vi "CV.vi"(2 "Run uninterrupted?":bool, 3 "Device Category IN:":string(combo)="ATLAS18SS" caption="Device Category:", 4 "Batch No. IN:":string caption="Batch No.:", 5 "Wafer No. IN:":string caption="Wafer No.:", 6 "DB Serial No. IN:":string caption="DB Serial No.:") -> (0 "Done!":bool)   [LabVIEW 2013]
doc: "Performs CV measurements according to ATLAS ITk Quality Control Specifications."
uses:
  InstrControl/Switching/Switching.lvclass
  InstrControl/SupplyControl/SupplyControl.lvclass
  InstrControl/LCRControl/LCRControl.lvclass
  general_VIs/globals/QC_MeasurementSetup.vi
  general_VIs/globals/QC_RunInformation.vi
  InstrControl/InstrumentSetup.vi
  InstrControl/ArduinoControl/ArduinoControl.lvclass
  <vilib>/Analysis/NI_AALBase.lvlib
  InstrControl/InstrControl.lvclass
panel:
  out "Tab Control 2":enum32{"CV Setup", "CV Scan"}(tab)
  in  "V_depletion limit [V]":dbl=-300.0
  in  "step interval [s] IN":i32=5 caption="step interval [s]"
  in  "step [V] IN":dbl=10.0 caption="step [V]" format="%.1f"
  in  "Final volts [V] IN":dbl=-500.0 caption="Final volts [V]"
  in  "Initial volts [V] IN":dbl caption="Initial volts [V]"
  in  "Current Limit [µA]":dbl=1000.0 min=0.0001 format="%.3f"
  in  "Continue":bool
  in  "Quit":bool
  in  "Software current limit?":bool
  in  "Frequency [Hz] Setup":i32=500 caption="Frequency [Hz]" format="%#.3p"
  in  "Measurement Configurations":bool
  out "RH":dbl[](array[numeric]) caption="RH [%]" format="%#.2f"
  out "step interval [s]":u32=5
  out "step [V]":dbl=10.0 format="%.1f"
  out "Final volts [V]":dbl=-700.0 format="%.1f"
  out "Initial volts [V]":dbl format="%.1f"
  out "Frequency [Hz]":i32=1000 format="%#.3p"
  out "Temp.":dbl[](array[numeric]) caption="Temp. [°C]" format="%#.2f"
  out "Volts":dbl[](array[numeric]) caption="Volts [V]"
  out "Resistance":dbl[](array[numeric]) caption="Res [kOhm]"
  out "Capacitance":dbl[](array[numeric]) caption="Cap [pF]"
  out "Cgraph":cluster{"Initial volts":dbl, dbl, dbl[]}(graph)
  in  "Scales":T1(ring)
  in  "Cscale":enum16{"1/C^2 [1/nF^2]", "nF", "pF"}(ring)
  out "positive ramp?":bool
  out "Tab Control":enum32{"CV Setup", "CV Scan"}(tab)
  in  "LCR Meter":string(combo)="WayneKerr 6440B"
  in  "User:":string(combo)="Christoph"
  in  "CV Supply":string(combo)="Keithley 2410"
  in  "Hardware Configurations":bool
  in  "Temperature":enum16{"Read Arduino", "Enter manually"}(ring)
  in  "Manufacturer:":string(combo)="Hamamatsu"
  in  "abort":bool
  out "Device Category:":string
  out "DB Serial No.:":string
  out "Current Volts:":dbl format="%.2f"
  in  "quit (no save)":bool
  in  "Quit & Save":bool
  out "Bias On/Off:":bool
  out "STATUS 1":string
  out "Initiated:":string
  out "Sensor No.:":string
  out "No of steps":u32
  out "Current reading No.":u32
  out "Last reading at:":string
  in  "Simulation":bool
  # "Strip Sensor QC: CV"
  # "University of\nCambridge"
  # "Vertical Scale:"
  # "Measurement Configuration"
  # "CV Scan parameters:"
  # "Last 5 readings:"
  # "n-4"
  # "n-3"
  # "n-2"
  # "n-1"
  # "n"
  # "DUT Description"
  # "Hardware"
  # "DUT & Test Description:"
  # "Current status:"
  # "Rdg No:"
  # "out of"
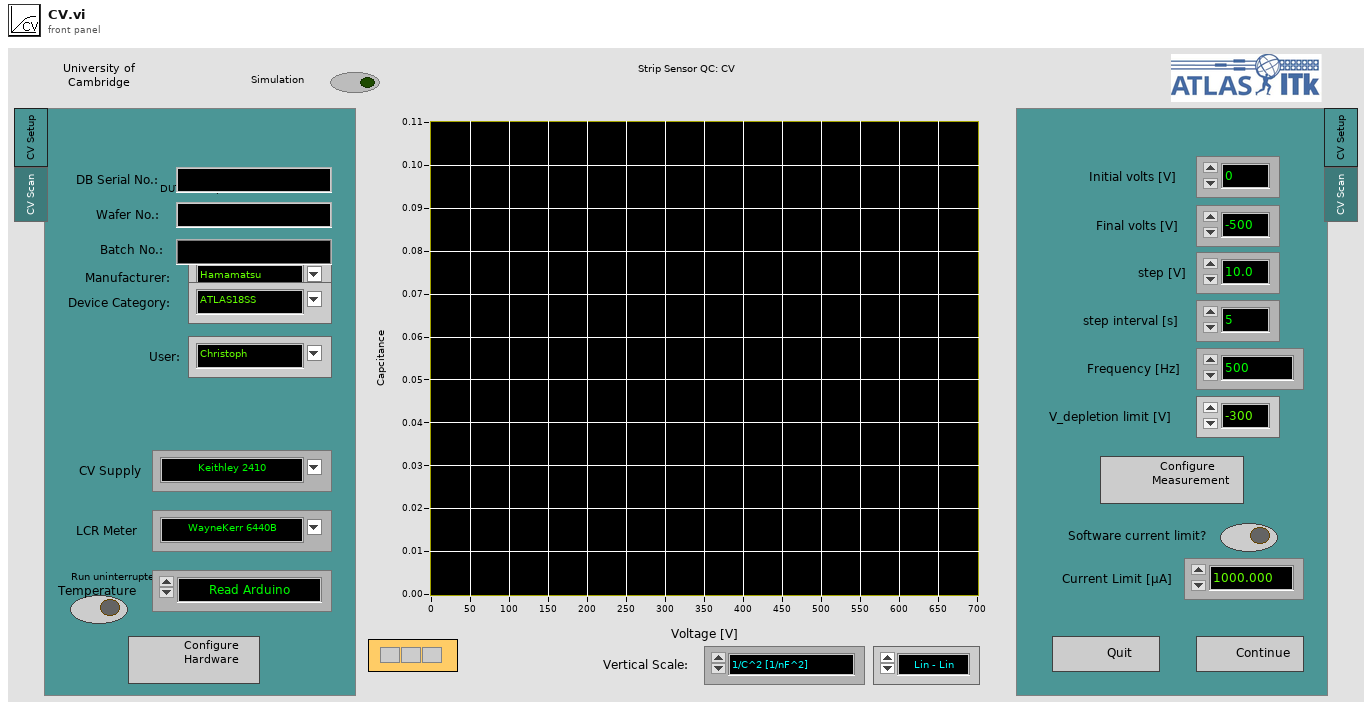
[diagram p1: front panel]
types:
  T1 = enum16{"Lin - Lin", "Log - Lin", "Lin - Log", "Log - log"}
  T2 = enum16{"Supply", "LCR", "Multimeter", "Switching"}
  T3 = enum16{"Reset", "Read Array", "Read Element", "Write Element", "Write Array", "Add Element", "Add Array"}
  T4 = enum16{"Reset", "Ground", "Striptest SMU", "Striptest LCR", "IV", "CV", "Interstrip Cap", "Interstrip Res"}
  T5 = enum32{"IV", "CV", "Stability", "Striptest", "Cis", "Ris", "PTP"}
  T6 = cluster{"Institute":string, "Manufacturers":string[], "Devices":string[], "Serialnumbers Lookup DB":string, "Data directory":string, "Backup & screenshot directory":string, "List of known users":string[], "Measurement switch not used":bool, "Measurement Switch":string, "DUT Switch":string, "Rseries IV [MOhm]":string, "Rshunt IV [MOhm]":string, "Rseries CV [MOhm]":string, "DC blocking Cap [µF]":string, "Rseries LCR [MOhm]":string, "Rseries stability [MOhm]":string, "Rshunt stability [MOhm]":string, "Rseries striptest bias [MOhm]":string, "Rseries strip pinhole [MOhm]":string}
  T7 = cluster{"Sensor Serial No.:":string, "Wafer:":string, "Batch:":string, "Manufacturer:":string, "Device Category:":string, "Database Serial No.:":string, "Date Initiated:":string, "Time Initiated:":string, "Test":string, "Probeplan used:":string, "End of Run comment:":string, "User:":string, "Vbias SMU":string, "LCR":string, "Test SMU":string, "Test DMM":string}
  T8 = cluster{"Supply":refnum<class "SupplyControl.lvclass">, "LCR":refnum<class "LCRControl.lvclass">, "Arduino":refnum<class "ArduinoControl.lvclass">, "Measurement switch":refnum<class "Switching.lvclass">, "Initial Voltage [V]":dbl, "Final Voltage [V]":dbl, "Step Size [V]":dbl, "Step Interval [s]":i32, "Number Of Steps":u32, "AC frequency [Hz]":i32, "RC Configuration":u16, "AC amplitude [V]":dbl, "Ramp down steps [V]":dbl, "Ramp down Interval [s]":i32, "Set Current Limit?":bool, "Current Limit [µA]":dbl, "Temperature Readout":enum16{"Read Arduino", "Enter manually"}, "Supply Name":string, "LCR Name":string, "V_depletion Limit [V]":dbl, "Measurement switch used?":bool}
  T9 = cluster{"VISA address":refnum<visa-resource-name>, "T sensor":enum16{"SHT", "DS"}, "Arduino":refnum<class "ArduinoControl.lvclass">}
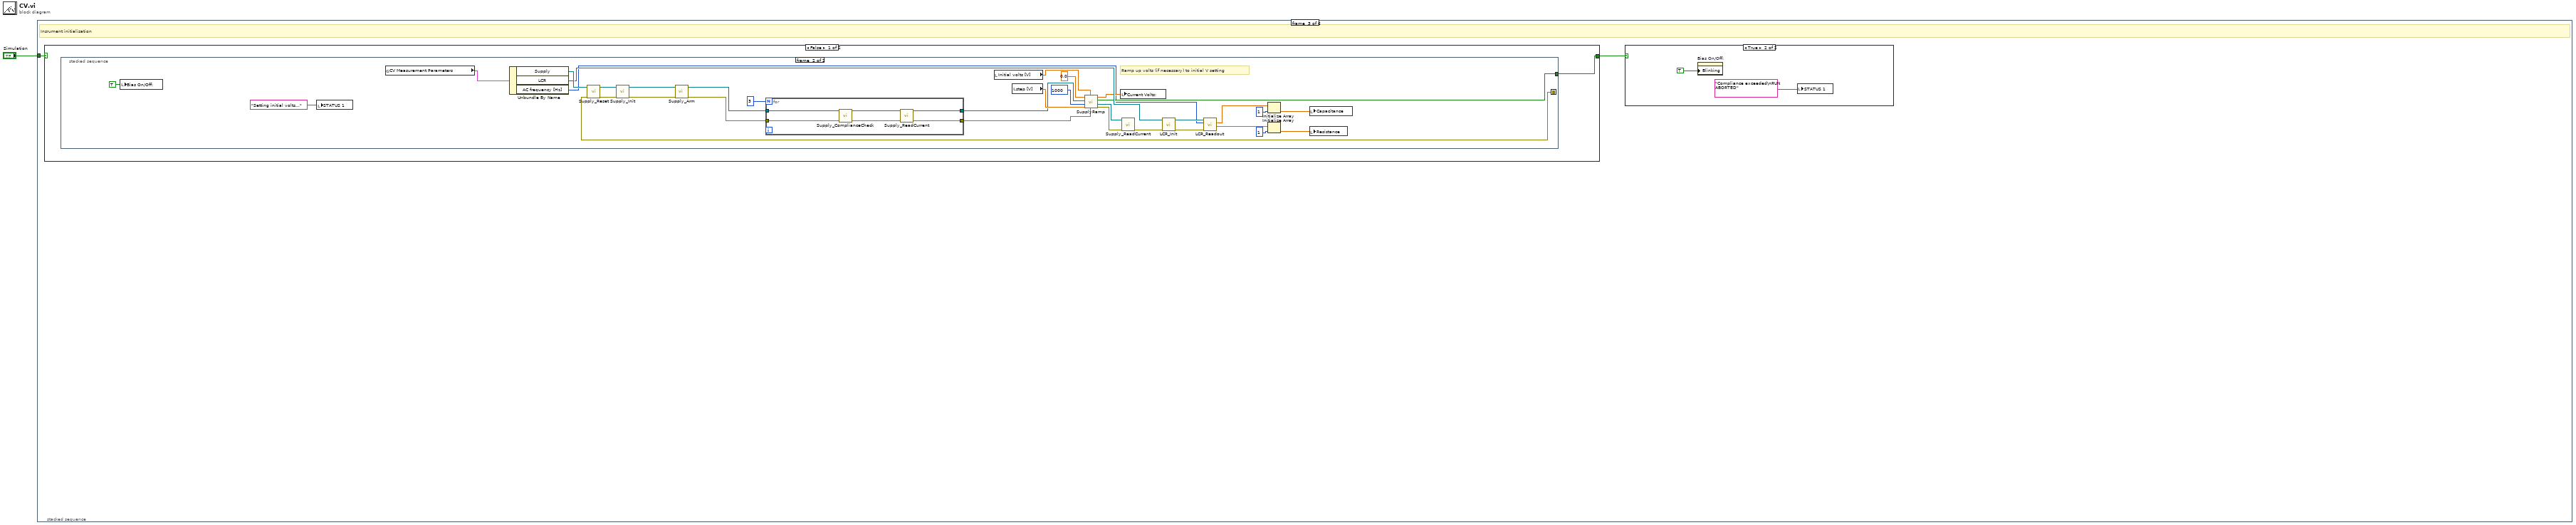
[diagram p0: block diagram]
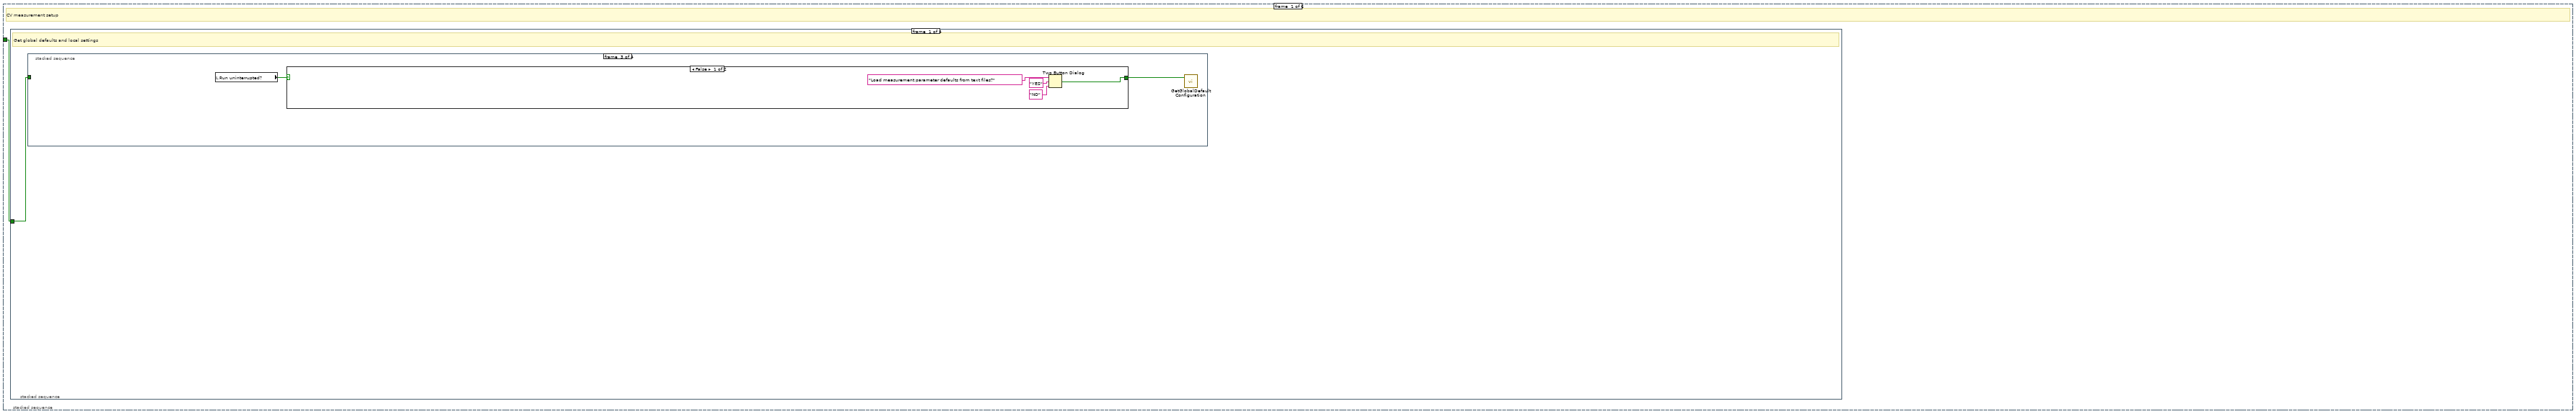
[diagram p2: hidden frame]
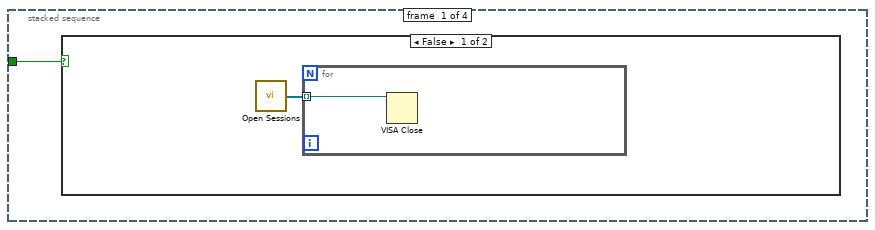
[diagram p3: hidden frame]
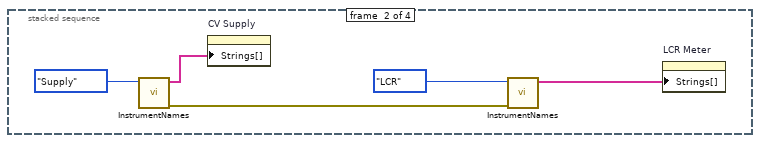
[diagram p5: hidden frame]
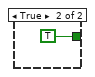
[diagram p6: hidden frame]
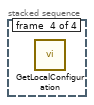
[diagram p7: hidden frame]
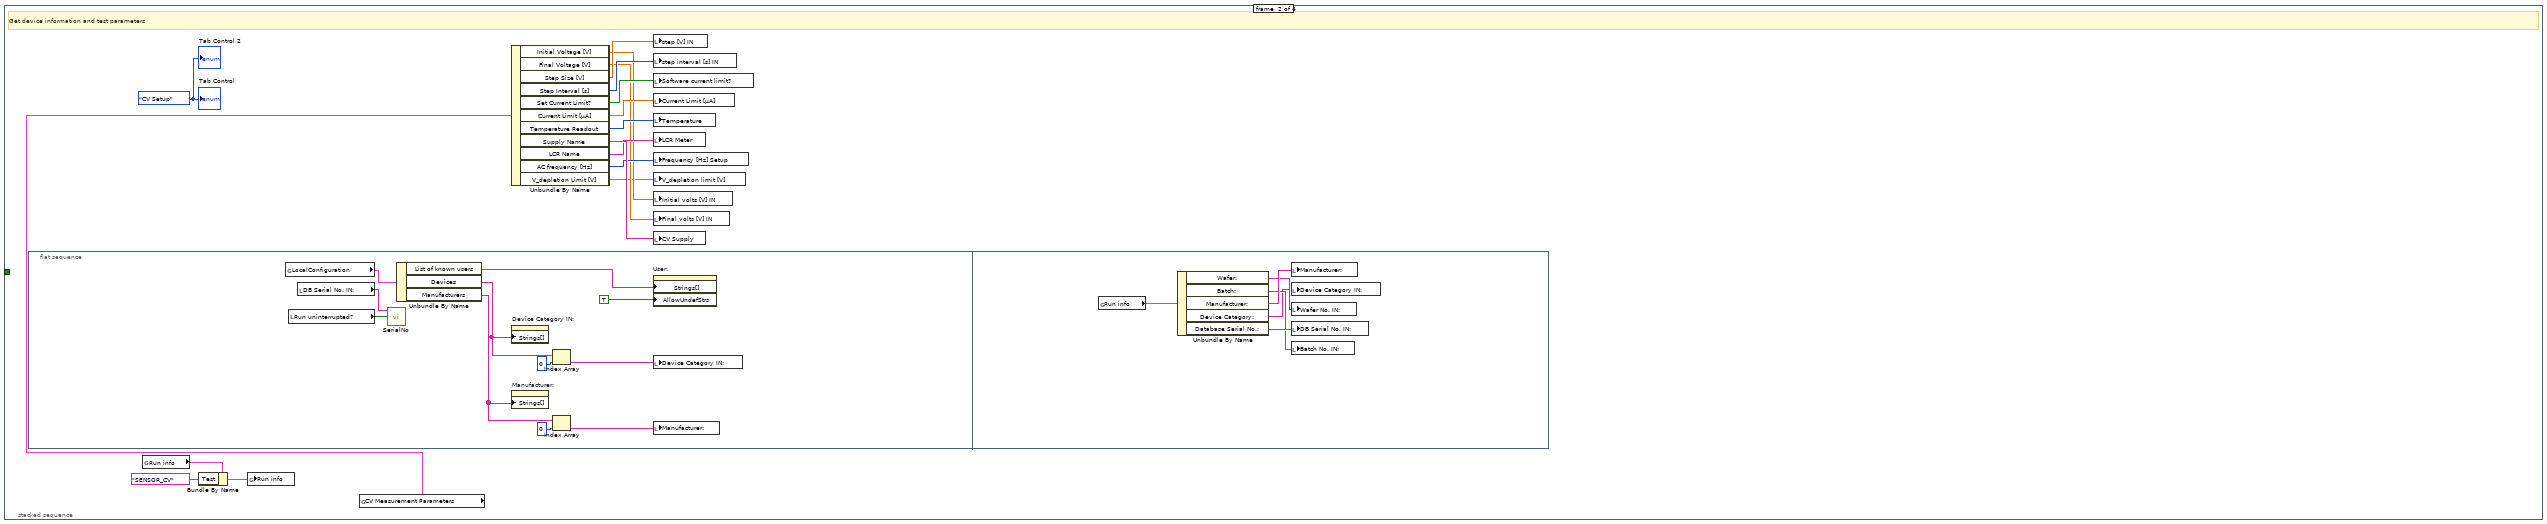
[diagram p8: hidden frame]
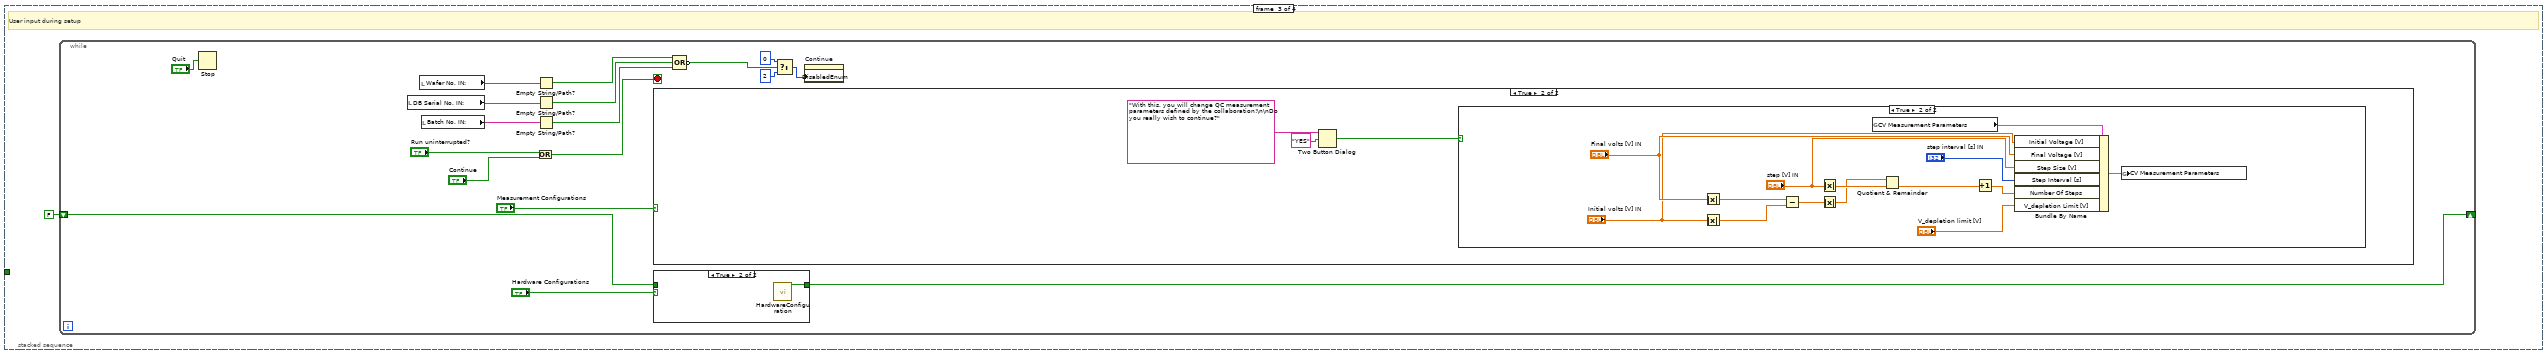
[diagram p9: hidden frame]
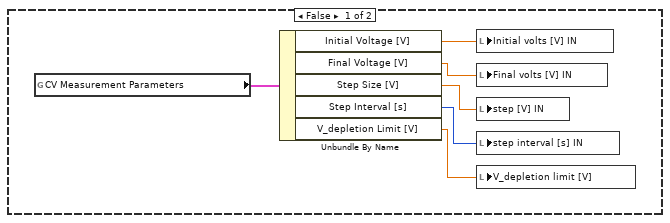
[diagram p12: hidden frame]
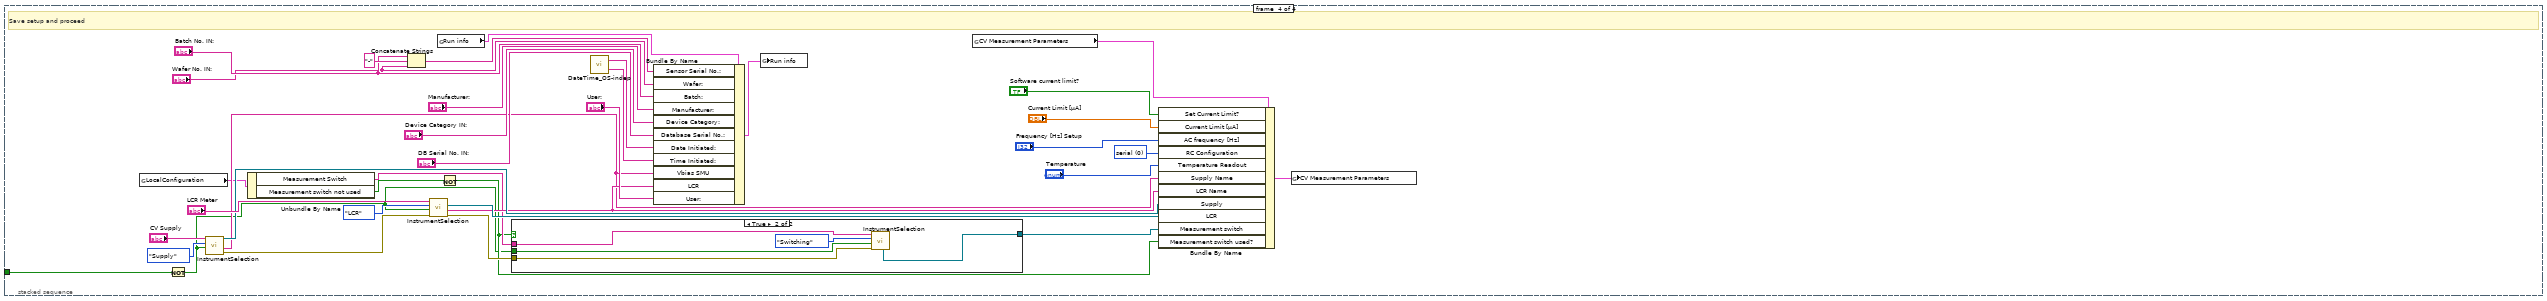
[diagram p13: hidden frame]
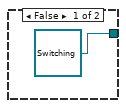
[diagram p14: hidden frame]
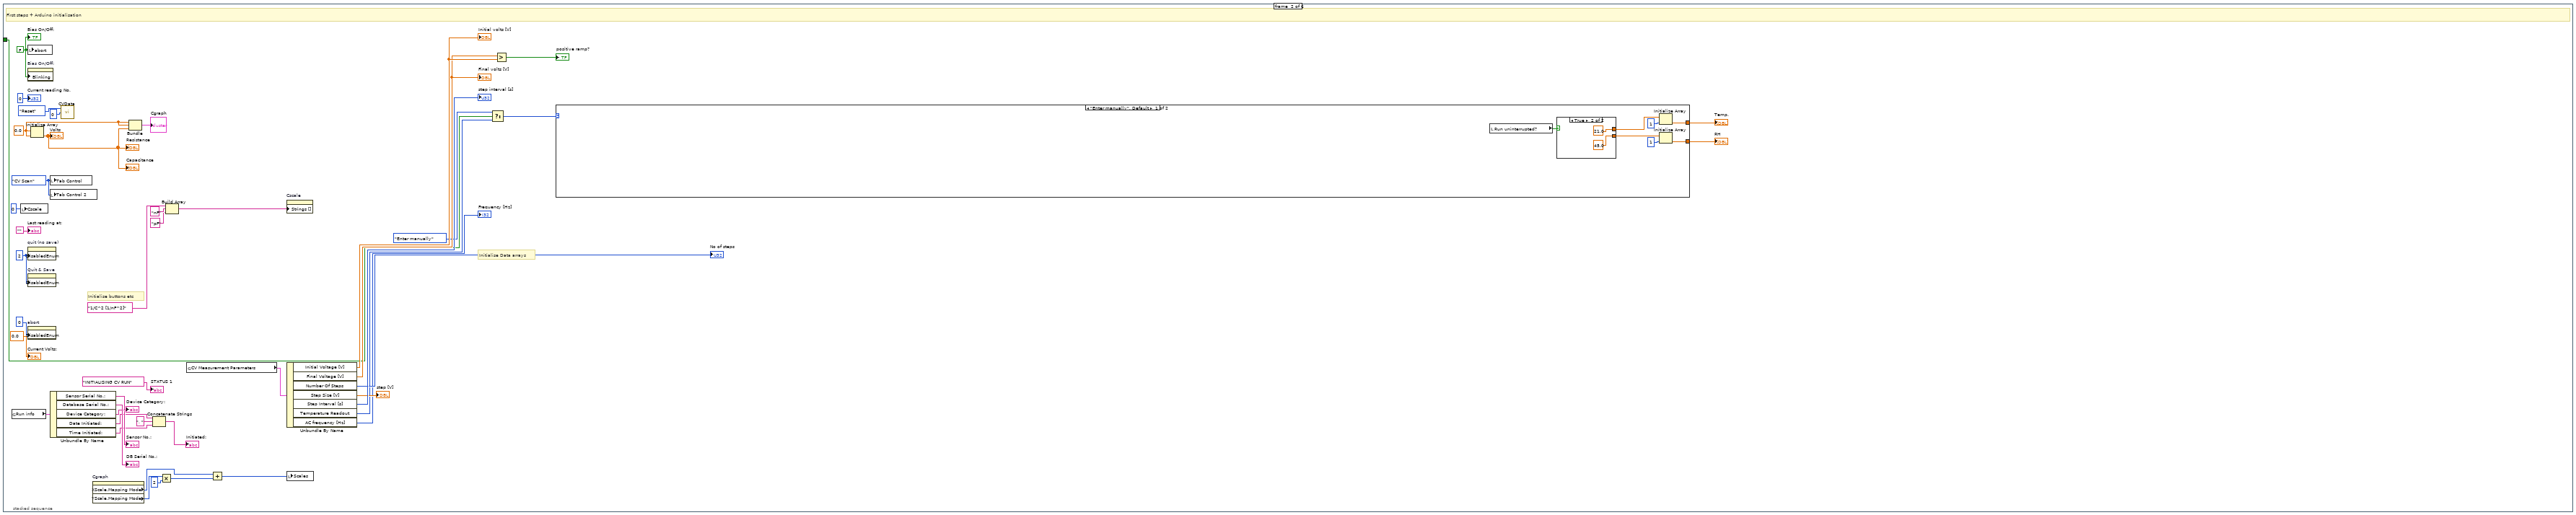
[diagram p15: hidden frame]
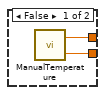
[diagram p16: hidden frame]
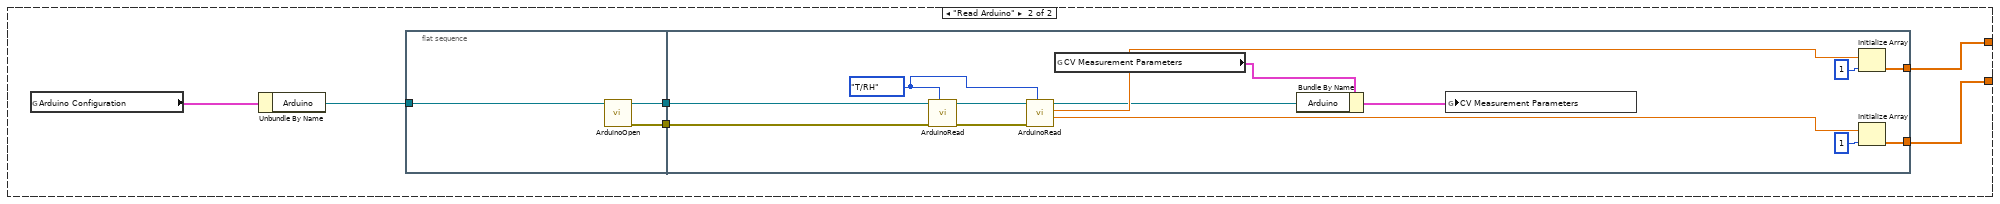
[diagram p17: hidden frame]
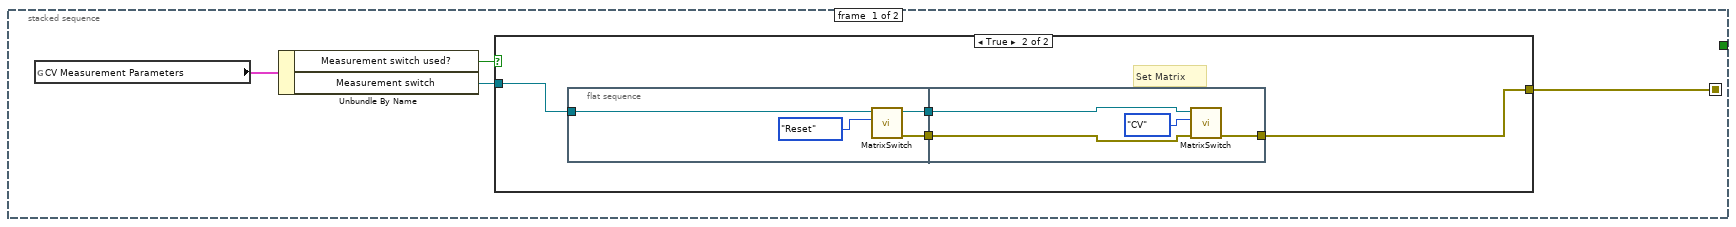
[diagram p18: hidden frame]
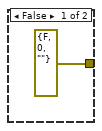
[diagram p19: hidden frame]
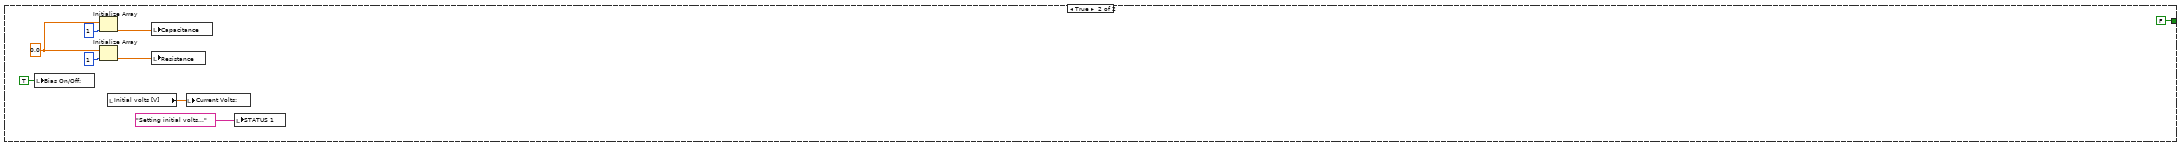
[diagram p20: hidden frame]
diagram:
  n1 = stacked-sequence {
    tunnel: "Simulation" -> [w2 w140 w217 w287 w615 w653]
    frame #0 {
      # "CV measurement setup"
      n2 = stacked-sequence {
        tunnel: w2 -> [w3 _ _ w99]
        frame #0 {
          # "Get global defaults and local settings"
          n3 = stacked-sequence {
            tunnel: w3 -> [w4 _ _ _]
            frame #0 {
              n4 = case shown="False" w4 {
                frame False {
                  n5 = call <vilib>:"Open Sessions.vi"() -> ("Array of Refnums"=w5:refnum<visa-resource-name>[])  [unwired: 2 in]
                  n6 = for {
                    tunnel: w5 -> [w6] mode=indexing
                    n7 = VISA Close(VISA resource name=w6) -> ()  [unwired: 1 in, 1 out]
                  }
                }
                frame True {
                }
              }
            }
            frame #1 {
              n8 = call "InstrumentNames.vi"("Instrument type"=T2."Supply") -> ("error out"=w11:errorcluster, "Instrument names"=w9:string[])  [unwired: 9 in]
              n9 = property on="CV Supply" class="CmbBox"("Strings[]"=w9) -> ()  [unwired: 2 in, 2 out]
              n10 = call "InstrumentNames.vi"("error in (no error)"=w11, "Instrument type"=T2."LCR") -> ("Instrument names"=w10:string[])  [unwired: 8 in, 1 out]
              n11 = property on="LCR Meter" class="CmbBox"("Strings[]"=w10) -> ()  [unwired: 2 in, 2 out]
            }
            frame #2 {
              n12 = local read "Run uninterrupted?"() -> (w13:bool)
              n13 = case shown="False" w13 {
                tunnel: [w16 TRUE] -> w12
                frame False {
                  n14 = Two Button Dialog(message="Load measurement parameter defaults from text files?", 1:"NO", 2:"YES") -> (T button?=w16:bool)
                }
                frame True {
                }
              }
              n15 = call "GetGlobalDefaultConfiguration.vi"("Read defaults?"=w12) -> ()  [unwired: 3 in]
            }
            frame #3 {
              n16 = call "GetLocalConfiguration.vi"() -> ()  [unwired: 3 in, 1 out]
            }
          }
        }
        frame #1 {
          w27 = enum32{"CV Setup", "CV Scan"}."CV Setup" ("Tab Control")
          # "Get device information and test parameters"
          n17 = flat-sequence {
            frame #0 {
              n18 = global read "QC_RunInformation.vi" "LocalConfiguration"() -> (w45:T6)
              n19 = local read "Run uninterrupted?"() -> (w42:bool)
              n20 = local read "DB Serial No. IN:"() -> (w35:string)
              n21 = call "SerialNo.vi"("DB serial number IN"=w35, "Run uninterrupted?"=w42) -> ()  [unwired: 6 in, 2 out]
              n22 = Unbundle By Name(w45) -> ("List of known users"=w44:string[], "Devices"=w38:string[], "Manufacturers"=w40:string[])
              n23 = property on="Device Category IN:" class="CmbBox"("Strings[]"=w38) -> ()  [unwired: 2 in, 2 out]
              n24 = property on="Manufacturer:" class="CmbBox"("Strings[]"=w40) -> ()  [unwired: 2 in, 2 out]
              n25 = Index Array(array=w38, index=0) -> (element=w37:string)
              n26 = Index Array(array=w40, index=0) -> (element=w36:string)
              n27 = property on="User:" class="CmbBox"("Strings[]"=w44, "AllowUndefStrs"=TRUE) -> ()  [unwired: 2 in, 2 out]
              n28 = local write "Device Category IN:"(w37) -> ()
              n29 = local write "Manufacturer:"(w36) -> ()
            }
            frame #1 {
              n30 = global read "QC_RunInformation.vi" "Run info"() -> (w51:T7)
              n31 = Unbundle By Name(w51) -> ("Wafer:"=w47:string, "Batch:"=w48:string, "Manufacturer:"=w49:string, "Device Category:"=w46:string, "Database Serial No.:"=w50:string)
              n32 = local write "Manufacturer:"(w49) -> ()
              n33 = local write "Device Category IN:"(w46) -> ()
              n34 = local write "Wafer No. IN:"(w47) -> ()
              n35 = local write "DB Serial No. IN:"(w50) -> ()
              n36 = local write "Batch No. IN:"(w48) -> ()
            }
          }
          n37 = global read "QC_RunInformation.vi" "Run info"() -> (w20:T7)
          n38 = Bundle By Name(cluster=w20, "Test"="SENSOR_CV") -> (w19:T7)
          n39 = global write "QC_RunInformation.vi" "Run info"(w19) -> ()
          n40 = global read "QC_MeasurementSetup.vi" "CV Measurement Parameters"() -> (w32:T8)
          n41 = Unbundle By Name(w32) -> ("Initial Voltage [V]"=w23:dbl, "Final Voltage [V]"=w24:dbl, "Step Size [V]"=w25:dbl, "Step Interval [s]"=w26:i32, "Set Current Limit?"=w31:bool, "Current Limit [µA]"=w30:dbl, "Temperature Readout"=w34:enum16{"Read Arduino", "Enter manually"}, "Supply Name"=w33:string, "LCR Name"=w29:string, "AC frequency [Hz]"=w28:i32, "V_depletion Limit [V]"=w22:dbl)
          n42 = local write "step [V] IN"(w25) -> ()
          n43 = local write "step interval [s] IN"(w26) -> ()
          n44 = local write "Software current limit?"(w31) -> ()
          n45 = local write "Current Limit [µA]"(w30) -> ()
          n46 = local write "Temperature"(w34) -> ()
          n47 = local write "LCR Meter"(w29) -> ()
          n48 = local write "Frequency [Hz] Setup"(w28) -> ()
          n49 = local write "V_depletion limit [V]"(w22) -> ()
          n50 = local write "Initial volts [V] IN"(w23) -> ()
          n51 = local write "Final volts [V] IN"(w24) -> ()
          n52 = local write "CV Supply"(w33) -> ()
          "Tab Control" <- w27
          "Tab Control 2" <- w27
        }
        frame #2 {
          # "User input during setup"
          n53 = while {
            shift-right: [w53] -> _
            shift-left: FALSE -> [w55]
            stop <- w57 stop-if-true
            n54 = Stop(stop? (T)="Quit") -> ()
            n55 = local read "DB Serial No. IN:"() -> (w68:string)
            n56 = local read "Wafer No. IN:"() -> (w69:string)
            n57 = local read "Batch No. IN:"() -> (w61:string)
            n58 = Or(x="Run uninterrupted?", y="Continue") -> (x .or. y?=w57:bool)
            n59 = Empty String/Path?(string/path=w69) -> (empty?=w66:bool)
            n60 = Empty String/Path?(string/path=w68) -> (empty?=w67:bool)
            n61 = Empty String/Path?(string/path=w61) -> (empty?=w60:bool)
            n62 = case shown="True" "Measurement Configurations" {
              frame False {
              }
              frame True {
                n63 = Two Button Dialog(message="With this, you will change QC measurement parameters defined by the collaboration!\n\nDo you really wish to continue?", 2:"YES") -> (T button?=w73:bool)  [unwired: 1 in]
                n64 = case shown="True" w73 {
                  frame False {
                    n65 = global read "QC_MeasurementSetup.vi" "CV Measurement Parameters"() -> (w81:T8)
                    n66 = Unbundle By Name(w81) -> ("Initial Voltage [V]"=w78:dbl, "Final Voltage [V]"=w77:dbl, "Step Size [V]"=w79:dbl, "Step Interval [s]"=w80:i32, "V_depletion Limit [V]"=w76:dbl)
                    n67 = local write "Initial volts [V] IN"(w78) -> ()
                    n68 = local write "Final volts [V] IN"(w77) -> ()
                    n69 = local write "step [V] IN"(w79) -> ()
                    n70 = local write "step interval [s] IN"(w80) -> ()
                    n71 = local write "V_depletion limit [V]"(w76) -> ()
                  }
                  frame True {
                    n72 = Absolute Value(x="Final volts [V] IN") -> (abs(x)=w87:dbl)
                    n73 = Absolute Value(x="Initial volts [V] IN") -> (abs(x)=w88:dbl)
                    n74 = Subtract(x=w87, y=w88) -> (x-y=w91:dbl)
                    n75 = Absolute Value(x="step [V] IN") -> (abs(x)=w90:dbl)
                    n76 = Absolute Value(x=w91) -> (abs(x)=w89:dbl)
                    n77 = global read "QC_MeasurementSetup.vi" "CV Measurement Parameters"() -> (w95:T8)
                    n78 = Quotient & Remainder(x=w89, y=w90) -> (floor(x/y)=w86:dbl)  [unwired: 1 out]
                    n79 = Increment(x=w86) -> (x+1=w85:dbl)
                    n80 = Bundle By Name(cluster=w95, "Initial Voltage [V]"="Initial volts [V] IN", "Final Voltage [V]"="Final volts [V] IN", "Step Size [V]"="step [V] IN", "Step Interval [s]"="step interval [s] IN", "Number Of Steps"=w85, "V_depletion Limit [V]"="V_depletion limit [V]") -> (w94:T8)
                    n81 = global write "QC_MeasurementSetup.vi" "CV Measurement Parameters"(w94) -> ()
                  }
                }
              }
            }
            n82 = case shown="True" "Hardware Configurations" {
              tunnel: [w71 w72] -> w53
              tunnel: w55 -> [w71 _]
              frame False {
              }
              frame True {
                n83 = call "HardwareConfiguration.vi"() -> ("configured?"=w72:bool)  [unwired: 11 in]
              }
            }
            n84 = Compound Arithmetic op=OR(w66, w67, w60) -> (invert w65:bool)
            n85 = Select(t=0, s=w65, f=2) -> (s? t:f=w62:i32)
            n86 = property on="Continue" class="Bool"("DisabledEnum"=w62) -> ()  [unwired: 2 in, 2 out]
          }
        }
        frame #3 {
          w122 = u16 0 items=["serial", "parallel"] ("RC Configuration")
          # "Save setup and proceed"
          n87 = global read "QC_RunInformation.vi" "LocalConfiguration"() -> (w104:T6)
          n88 = Not(x=w99) -> (.not. x?=w98:bool)
          n89 = call "InstrumentSelection.vi"("Verify GPIB address"=w98, "Instrument type"=T2."Supply", "Instrument name IN"="CV Supply") -> ("error out"=w118:errorcluster, "Instrument name OUT"=w106:string, "Supply"=w117:refnum<class "SupplyControl.lvclass">)  [unwired: 3 in, 3 out]
          n90 = Unbundle By Name(w104) -> ("Measurement Switch"=w102:string, "Measurement switch not used"=w103:bool)
          n91 = Concatenate Strings("Batch No. IN:", "-", "Wafer No. IN:") -> (w108:string)
          n92 = call "InstrumentSelection.vi"("error in (no error)"=w118, "Verify GPIB address"=w98, "Instrument type"=T2."LCR", "Instrument name IN"="LCR Meter") -> ("error out"=w105:errorcluster, "Instrument name OUT"=w107:string, "LCR"=w116:refnum<class "LCRControl.lvclass">)  [unwired: 2 in, 3 out]
          n93 = global read "QC_RunInformation.vi" "Run info"() -> (w127:T7)
          n94 = Not(x=w103) -> (.not. x?=w101:bool)
          n95 = case shown="True" w101 {
            tunnel: w105 -> [_ w136]
            tunnel: [refnum<class "Switching.lvclass"> refnum ("Switching") w135] -> w100
            tunnel: w98 -> [_ w134]
            tunnel: w102 -> [_ w133]
            frame False {
            }
            frame True {
              n96 = call "InstrumentSelection.vi"("error in (no error)"=w136, "Verify GPIB address"=w134, "Instrument type"=T2."Switching", "Instrument name IN"=w133) -> ("Switching"=w135:refnum<class "Switching.lvclass">)  [unwired: 2 in, 5 out]
            }
          }
          n97 = call "DateTime_OS-indep.vi"() -> ("Time"=w96:string, "Date"=w97:string)
          n98 = Bundle By Name(cluster=w127, "Sensor Serial No.:"=w108, "Wafer:"="Wafer No. IN:", "Batch:"="Batch No. IN:", "Manufacturer:"="Manufacturer:", "Device Category:"="Device Category IN:", "Database Serial No.:"="DB Serial No. IN:", "Date Initiated:"=w97, "Time Initiated:"=w96, "Vbias SMU"=w106, "LCR"=w107, "User:"="User:") -> (w126:T7)
          n99 = global write "QC_RunInformation.vi" "Run info"(w126) -> ()
          n100 = global read "QC_MeasurementSetup.vi" "CV Measurement Parameters"() -> (w130:T8)
          n101 = Bundle By Name(cluster=w130, "Set Current Limit?"="Software current limit?", "Current Limit [µA]"="Current Limit [µA]", "AC frequency [Hz]"="Frequency [Hz] Setup", "RC Configuration"=w122, "Temperature Readout"="Temperature", "Supply Name"=w106, "LCR Name"=w107, "Supply"=w117, "LCR"=w116, "Measurement switch"=w100, "Measurement switch used?"=w101) -> (w131:T8)
          n102 = global write "QC_MeasurementSetup.vi" "CV Measurement Parameters"(w131) -> ()
        }
      }
    }
    frame #1 {
      w148 = enum32{"CV Setup", "CV Scan"}."CV Scan" ("Tab Control")
      w165 = 2
      w171 = 0.0
      w164 = FALSE ("Visible")
      # "Initialise buttons etc"
      # "Initialise Data arrays"
      # "First steps + Arduino initialisation"
      n103 = global read "QC_RunInformation.vi" "Run info"() -> (w181:T7)
      n104 = local write "Cscale"(u16 0 ("Scale")) -> ()
      n105 = local write "abort"(w164) -> ()
      n106 = property on="Bias On/Off:" class="Bool (strict)"("Blinking"=w164) -> ()  [unwired: 2 in, 2 out]
      n107 = property on="quit (no save)" class="Bool"("DisabledEnum"=w165) -> ()  [unwired: 2 in, 2 out]
      n108 = property on="Quit & Save" class="Bool"("DisabledEnum"=w165) -> ()  [unwired: 2 in, 2 out]
      n109 = property on="abort" class="Bool (strict)"("DisabledEnum"=0) -> ()  [unwired: 2 in, 2 out]
      n110 = Initialize Array(w171, w171) -> (w150:dbl[])
      "Volts" <- w150
      "Capacitance" <- w150
      "Resistance" <- w150
      n111 = local write "Tab Control"(w148) -> ()
      n112 = local write "Tab Control 2"(w148) -> ()
      n113 = Unbundle By Name(w181) -> ("Sensor Serial No.:"=→"Sensor No.:":string, "Database Serial No.:"=→"DB Serial No.:":string, "Device Category:"=→"Device Category:":string, "Date Initiated:"=w145:string, "Time Initiated:"=w143:string)
      n114 = call "CVData.vi"("Action"=T3."Reset", "Array Size / Index"=0) -> ()  [unwired: 3 in, 2 out]
      n115 = property on="Cgraph" class="WFGraph (strict)"() -> ("XScale.Mapping Mode"=w157:u8, "YScale.Mapping Mode"=w156:u8)  [unwired: 2 in, 2 out]
      n116 = Bundle(w171, w171, w150) -> (→"Cgraph":cluster{dbl, dbl, dbl[]})  [unwired: 1 in]
      n117 = Concatenate Strings(w145, ", ", w143) -> (→"Initiated:":string)
      n118 = Multiply(x=w156, y=2) -> (x*y=w159:i32)
      n119 = Build Array("1/C^2 [1/nF^2]", "nF", "pF") -> (w178:string[])
      n120 = global read "QC_MeasurementSetup.vi" "CV Measurement Parameters"() -> (w153:T8)
      n121 = Add(x=w157, y=w159) -> (x+y=w155:i32)
      n122 = property on="Cscale" class="Enum (strict)"("Strings []"=w178) -> ()  [unwired: 2 in, 2 out]
      n123 = Unbundle By Name(w153) -> ("Initial Voltage [V]"=w163:dbl, "Final Voltage [V]"=w162:dbl, "Number Of Steps"=→"No of steps":u32, "Step Size [V]"=→"step [V]":dbl, "Step Interval [s]"=→"step interval [s]":i32, "Temperature Readout"=w138:enum16{"Read Arduino", "Enter manually"}, "AC frequency [Hz]"=→"Frequency [Hz]":i32)
      "Initial volts [V]" <- w163
      "Final volts [V]" <- w162
      n124 = local write "Scales"(w155) -> ()
      n125 = Select(t=enum16{"Read Arduino", "Enter manually"}."Enter manually" ("Temperature Readout"), s=w140, f=w138) -> (s? t:f=w139:enum16{"Read Arduino", "Enter manually"})
      n126 = Greater?(x=w162, y=w163) -> (0:→"positive ramp?":bool)
      n127 = case shown="\"Enter manually\", Default" w139 {
        tunnel: [w189 w199] -> w168
        tunnel: [w186 w198] -> w154
        frame "Enter manually", Default {
          n128 = local read "Run uninterrupted?"() -> (w183:bool)
          n129 = case shown="True" w183 {
            tunnel: [w191 21.0] -> w185
            tunnel: [w190 45.0] -> w184
            frame False {
              n130 = call "ManualTemperature.vi"() -> ("Humidity [%] out"=w190:dbl, "Temperature [°C] out"=w191:dbl)
            }
            frame True {
            }
          }
          n131 = Initialize Array(w185, 1) -> (w189:dbl[])
          n132 = Initialize Array(w184, 1) -> (w186:dbl[])
        }
        frame "Read Arduino" {
          n133 = global read "InstrumentSetup.vi" "Arduino Configuration"() -> (w195:T9)
          n134 = Unbundle By Name(w195) -> ("Arduino"=w194:refnum<class "ArduinoControl.lvclass">)
          n135 = flat-sequence {
            tunnel: [w200] -> w197
            tunnel: [w202] -> w196
            tunnel: w194 -> [w201]
            tunnel: [w216] -> w199
            tunnel: [w213] -> w198
            tunnel: w197 -> [w205]
            tunnel: w196 -> [w206]
            frame #0 {
              n136 = call "ArduinoOpen.vi"("ArduinoControl in"=w201) -> ("error out"=w202:errorcluster, "ArduinoControl out"=w200:refnum<class "ArduinoControl.lvclass">)  [unwired: 9 in]
            }
            frame #1 {
              w207 = enum16{"T/RH", "Interlock", "Edgesense"}."T/RH" ("Arduino function")
              n137 = call "ArduinoRead.vi"("Arduino function"=w207, "error in (no error)"=w206, "ArduinoControl in"=w205) -> ("error out"=w203:errorcluster, "ArduinoControl out"=w204:refnum<class "ArduinoControl.lvclass">)  [unwired: 3 in, 4 out]
              n138 = call "ArduinoRead.vi"("Arduino function"=w207, "error in (no error)"=w203, "ArduinoControl in"=w204) -> ("rel. Humidity [%]"=w211:dbl, "Temperature [°C]"=w212:dbl, "ArduinoControl out"=w210:refnum<class "ArduinoControl.lvclass">)  [unwired: 3 in, 3 out]
              n139 = global read "QC_MeasurementSetup.vi" "CV Measurement Parameters"() -> (w209:T8)
              n140 = Bundle By Name(cluster=w209, "Arduino"=w210) -> (w208:T8)
              n141 = global write "QC_MeasurementSetup.vi" "CV Measurement Parameters"(w208) -> ()
              n142 = Initialize Array(w212, 1) -> (w216:dbl[])
              n143 = Initialize Array(w211, 1) -> (w213:dbl[])
            }
          }
        }
      }
      "Temp." <- w168
      "RH" <- w154
      "STATUS 1" <- "INITIALISING CV RUN"
      "Bias On/Off:" <- w164
      "Last reading at:" <- ""
      "Current reading No." <- u32 0 ("Current reading No.")
      "Current Volts:" <- 0.0 ("Current Volts:")
    }
    frame #2 {
      # "Insrument initialisation"
      n144 = case shown="False" w217 {
        tunnel: [w219 FALSE] -> w218
        frame False {
          n145 = stacked-sequence {
            seq-local: [w221 _] -> [_ w249]
            tunnel: [_ w251] -> w219
            frame #0 {
              n146 = global read "QC_MeasurementSetup.vi" "CV Measurement Parameters"() -> (w220:T8)
              n147 = Unbundle By Name(w220) -> ("Measurement switch used?"=w223:bool, "Measurement switch"=w222:refnum<class "Switching.lvclass">)
              n148 = case shown="True" w223 {
                tunnel: w222 -> [_ w225]
                tunnel: [errorcluster {"status"=FALSE, "code"=0, "source"=""} ("error constant") w226] -> w221
                frame False {
                }
                frame True {
                  # "Set Matrix"
                  n149 = flat-sequence {
                    tunnel: [w232] -> w228
                    tunnel: [w231] -> w227
                    tunnel: w225 -> [w229]
                    tunnel: w228 -> [w236]
                    tunnel: w227 -> [w235]
                    tunnel: [w234] -> w226
                    frame #0 {
                      n150 = call-dynamic "MatrixSwitch.vi"("Action"=T4."Reset", "Switching in"=w229) -> ("error out"=w232:errorcluster, "Switching out"=w231:refnum<class "Switching.lvclass">)  [unwired: 7 in, 1 out]
                    }
                    frame #1 {
                      n151 = call-dynamic "MatrixSwitch.vi"("error in (no error)"=w236, "Action"=T4."CV", "Switching in"=w235) -> ("error out"=w234:errorcluster)  [unwired: 6 in, 2 out]
                    }
                  }
                }
              }
            }
            frame #1 {
              # "Ramp up volts (if necessary) to initial V setting"
              n152 = local write "Bias On/Off:"(TRUE ("Compliance?")) -> ()
              n153 = local write "STATUS 1"("Setting initial volts..." ("STATUS 1")) -> ()
              n154 = global read "QC_MeasurementSetup.vi" "CV Measurement Parameters"() -> (w265:T8)
              n155 = Unbundle By Name(w265) -> ("Supply"=w262:refnum<class "SupplyControl.lvclass">, "LCR"=w261:refnum<class "LCRControl.lvclass">, "AC frequency [Hz]"=w242:i32)
              n156 = call-dynamic "Supply_Reset.vi"("error in (no error)"=w249, "SupplyControl in"=w262) -> ("error out"=w267:errorcluster, "SupplyControl out"=w269:refnum<class "SupplyControl.lvclass">)  [unwired: 8 in]
              n157 = call-dynamic "Supply_Init.vi"("error in (no error)"=w267, "SupplyControl in"=w269) -> ("error out"=w266:errorcluster, "SupplyControl out"=w268:refnum<class "SupplyControl.lvclass">)  [unwired: 8 in]
              n158 = call-dynamic "Supply_Arm.vi"("error in (no error)"=w266, "SupplyControl in"=w268) -> ("error out"=w237:errorcluster, "SupplyControl out"=w241:refnum<class "SupplyControl.lvclass">)  [unwired: 8 in]
              n159 = for {
                N: 3 -> [_]
                tunnel: w241 -> [w273]
                tunnel: [w275] -> w240
                tunnel: [w274] -> w239
                tunnel: w237 -> [w271]
                n160 = call-dynamic "Supply_ComplianceCheck.vi"("error in (no error)"=w271, "SupplyControl in"=w273) -> ("error out"=w270:errorcluster, "SupplyControl out"=w272:refnum<class "SupplyControl.lvclass">)  [unwired: 6 in, 2 out]
                n161 = call-dynamic "Supply_ReadCurrent.vi"("error in (no error)"=w270, "SupplyControl in"=w272) -> ("error out"=w274:errorcluster, "SupplyControl out"=w275:refnum<class "SupplyControl.lvclass">)  [unwired: 7 in, 1 out]
              }
              n162 = local read "Initial volts [V]"() -> (w254:dbl)
              n163 = local read "step [V]"() -> (w255:dbl)
              n164 = call "SupplyRamp.vi"("error in"=w239, "Requested Voltage"=w254, "Step Size"=w255, "Step Delay"=1000, "Supply IN"=w240, "Starting Voltage"=0.0) -> ("error out"=w252:errorcluster, "Supply OUT"=w253:refnum<class "SupplyControl.lvclass">, "Compliance exceeded"=w251:bool, "Current Voltage"=w258:dbl)  [unwired: 2 in]
              n165 = local write "Current Volts:"(w258) -> ()
              n166 = call-dynamic "Supply_ReadCurrent.vi"("error in (no error)"=w252, "SupplyControl in"=w253) -> ("error out"=w250:errorcluster)  [unwired: 7 in, 2 out]
              n167 = call-dynamic "LCR_Init.vi"("error in (no error)"=w250, "LCRControl in"=w261) -> ("error out"=w247:errorcluster, "LCRControl out"=w248:refnum<class "LCRControl.lvclass">)  [unwired: 8 in]
              n168 = call-dynamic "LCR_Readout.vi"("error in (no error)"=w247, "Frequency in Hz"=w242, "LCRControl in"=w248) -> ("Resistance in Ohm"=w244:dbl, "Capacitance in pF"=w246:dbl)  [unwired: 5 in, 2 out]
              n169 = Initialize Array(w246, 1) -> (w259:dbl[])
              n170 = Initialize Array(w244, 1) -> (w243:dbl[])
              n171 = local write "Capacitance"(w259) -> ()
              n172 = local write "Resistance"(w243) -> ()
            }
          }
        }
        frame True {
          w277 = 0.0
          n173 = local write "Bias On/Off:"(TRUE ("Compliance?")) -> ()
          n174 = Initialize Array(w277, 1) -> (w280:dbl[])
          n175 = Initialize Array(w277, 1) -> (w278:dbl[])
          n176 = local read "Initial volts [V]"() -> (w284:dbl)
          n177 = local write "Capacitance"(w280) -> ()
          n178 = local write "Resistance"(w278) -> ()
          n179 = local write "Current Volts:"(w284) -> ()
          n180 = local write "STATUS 1"("Setting initial volts..." ("STATUS 1")) -> ()
        }
      }
      n181 = case shown="True" w218 {
        frame False {
        }
        frame True {
          n182 = property on="Bias On/Off:" class="Bool (strict)"("Blinking"=TRUE) -> ()  [unwired: 2 in, 2 out]
          n183 = local write "STATUS 1"("Compliance exceeded\nRUN ABORTED") -> ()
        }
      }
    }
    frame #3 {
      # "Initial compliance exceeded?"
      # "Measurement procedure"
      n184 = property on="Bias On/Off:" class="Bool (strict)"() -> ("Blinking"=w298:bool)  [unwired: 2 in, 2 out]
      n185 = case shown="False" w298 {
        tunnel: [w307 w612] -> w297
        tunnel: w287 -> [w304 _]
        frame False {
          n186 = while {
            shift-left: "Cscale" -> [w318]
            shift-right: [w317] -> _
            shift-left: "Scales" -> [w319]
            shift-right: [w320] -> _
            tunnel: [w316] -> w307
            tunnel: w304 -> [w308]
            stop <- w321 continue-if-true
            # "Main measurement loop"
            # "End of loop?"
            # "Compliance?"
            # "Main measurement loop. execute this if compliance ok after first setting initial volts"
            n187 = local read "step interval [s]"() -> (w313:u32)
            n188 = local read "Final volts [V]"() -> (w314:dbl)
            n189 = local read "step [V]"() -> (w315:dbl)
            n190 = stacked-sequence {
              tunnel: [w335 _] -> w320
              tunnel: w315 -> [w332 w405]
              tunnel: [_ w404] -> w310
              tunnel: w314 -> [_ w403]
              tunnel: w313 -> [w323 w402]
              tunnel: [_ w401] -> w312
              tunnel: w319 -> [w334 _]
              tunnel: w318 -> [w333 _]
              tunnel: [w331 _] -> w317
              tunnel: [_ w399] -> w311
              tunnel: w308 -> [_ w398]
              frame #0 {
                n191 = Format Into String(format string="%d", w323) -> (resulting string=w328:string)  [unwired: 2 in, 1 out]
                n192 = Get Date/Time In Seconds() -> (seconds since 1Jan1904=w325:timestamp)
                n193 = To Double Precision Float(number=w325) -> (double precision float=w326:dbl)
                n194 = Concatenate Strings("Waiting for  ", w328, " seconds...") -> (w324:string)
                n195 = while {
                  tunnel: w332 -> [w348]
                  shift-left: w333 -> [w352]
                  shift-right: [w345] -> w331
                  shift-left: w334 -> [w353]
                  shift-right: [w354] -> w335
                  tunnel: w324 -> [w346]
                  tunnel: w323 -> [w358]
                  tunnel: w326 -> [w359]
                  i -> [w338]
                  stop <- w360 continue-if-true
                  n196 = Absolute Value(x=w348) -> (abs(x)=w347:dbl)
                  n197 = Wait (ms)(milliseconds to wait=u32 100) -> ()  [unwired: 1 out]
                  n198 = Get Date/Time In Seconds() -> (seconds since 1Jan1904=w344:timestamp)
                  n199 = Quotient & Remainder(x=w338, y=10) -> (x-y*floor(x/y)=w337:i32)  [unwired: 1 out]
                  n200 = local read "Cscale"() -> (w345:enum16{"1/C^2 [1/nF^2]", "nF", "pF"})
                  n201 = local read "Scales"() -> (w354:T1)
                  n202 = To Double Precision Float(number=w344) -> (double precision float=w364:dbl)
                  n203 = Equal To 0?(x=w337) -> (x = 0?=w336:bool)
                  n204 = case shown="True" w336 {
                    frame False {
                    }
                    frame True {
                      n205 = global read "QC_MeasurementSetup.vi" "CV Measurement Parameters"() -> (w365:T8)
                      n206 = Unbundle By Name(w365) -> ("Supply"=w366:refnum<class "SupplyControl.lvclass">)
                      n207 = call-dynamic "Supply_ReadCurrent.vi"("SupplyControl in"=w366) -> ()  [unwired: 8 in, 3 out]
                    }
                  }
                  n208 = Not Equal?(x=w352, y=w345) -> (x != y?=w343:bool)
                  n209 = Not Equal?(x=w353, y=w354) -> (x != y?=w355:bool)
                  n210 = Subtract(x=w364, y=w359) -> (x-y=w341:dbl)
                  n211 = case shown="True" w343 {
                    tunnel: w347 -> [_ w378]
                    tunnel: w345 -> [_ w371]
                    frame False {
                    }
                    frame True {
                      n212 = local read "Current reading No."() -> (w376:u32)
                      n213 = property on="Cgraph" class="WFGraph (strict)"() -> ("YScale.Mapping Mode"=w373:u8)  [unwired: 2 in, 2 out]
                      n214 = call "CVData.vi"("Action"=T3."Read Array", "Array No."=u32 1 ("Action")) -> ("Array OUT"=w367:dbl[])  [unwired: 3 in, 1 out]
                      n215 = property on="Cgraph" class="WFGraph (strict)"("YScale.Minimum"=w373) -> ()  [unwired: 2 in, 2 out]
                      n216 = Array Subset(array=w367, index=0, length=w376) -> (w374:dbl[])
                      n217 = Absolute Value(x=w374) -> (abs(x)=w372:dbl[])
                      n218 = case shown="..\"1/C^2 [1/nF^2]\"" w371 {
                        tunnel: [w382 w385 w388] -> w370
                        tunnel: w372 -> [w380 w387 w388]
                        frame .."1/C^2 [1/nF^2]" {
                          n219 = Array Size(array=w380) -> (size(s)=w381:i32)
                          n220 = for {
                            N: w381 -> [_]
                            tunnel: w380 -> [w384] mode=indexing
                            tunnel: [w383] -> w382 mode=indexing
                            n221 = formula code="y=1000000./(x*x);"("x"=w384) -> ("y"=w383:dbl)
                          }
                        }
                        frame "nF" {
                          n222 = Divide(x=w387, y=1000.0) -> (x/y=w385:dbl[])
                        }
                        frame "pF".. {
                        }
                      }
                      n223 = local read "Initial volts [V]"() -> (w377:dbl)
                      n224 = Bundle("Initial volts [V]"=w377, w378, w370) -> (w375:cluster{"Initial volts [V]":dbl, dbl, dbl[]})  [unwired: 1 in]
                      n225 = local write "Cgraph"(w375) -> ()
                    }
                  }
                  n226 = case shown="True" w355 {
                    tunnel: w354 -> [_ w391]
                    frame False {
                    }
                    frame True {
                      n227 = case shown="\"Log - log\".." w391 {
                        tunnel: [w392 1 0 w397] -> w390
                        tunnel: [w392 0 1 w397] -> w389
                        frame .."Lin - Lin" {
                          w392 = 0
                        }
                        frame "Log - Lin" {
                        }
                        frame "Lin - Log" {
                        }
                        frame "Log - log".. {
                          w397 = 1
                        }
                      }
                      n228 = property on="Cgraph" class="WFGraph (strict)"("X Scale.Mapping Mode"=w390) -> ()  [unwired: 2 in, 2 out]
                      n229 = property on="Cgraph" class="WFGraph (strict)"("Y Scale.Mapping Mode"=w389, "YScale.Minimum"=w389) -> ()  [unwired: 2 in, 2 out]
                    }
                  }
                  n230 = Subtract(x=w358, y=w341) -> (x-y=w340:dbl)
                  n231 = local read "abort"() -> (w357:bool)
                  n232 = Not(x=w357) -> (.not. x?=w363:bool)
                  n233 = Greater Than 0?(x=w340) -> (x > 0?=w342:bool)
                  n234 = Format Into String(format string="%d", w340) -> (resulting string=w362:string)  [unwired: 2 in, 1 out]
                  n235 = And(x=w342, y=w363) -> (x .and. y?=w360:bool)
                  n236 = Concatenate Strings(w346, "\r\n", "Timer status: ", w362) -> (w356:string)
                  n237 = local write "STATUS 1"(w356) -> ()
                }
              }
              frame #1 {
                n238 = local read "abort"() -> (w400:bool)
                n239 = case shown="False" w400 {
                  tunnel: [w412 w609] -> w401
                  tunnel: w402 -> [w411 _]
                  tunnel: w403 -> [w410 _]
                  tunnel: [w408 w609] -> w404
                  tunnel: w405 -> [w409 _]
                  tunnel: [w407 w609] -> w399
                  tunnel: w398 -> [w406 _]
                  frame False {
                    n240 = stacked-sequence {
                      seq-local: [w438 _ _] -> [_ w499 _]
                      seq-local: [w437 _ _] -> [_ _ w567]
                      seq-local: [w425 _ _] -> [_ _ w568]
                      tunnel: w409 -> [_ w511 w573]
                      tunnel: w410 -> [_ _ w564]
                      tunnel: [_ _ w571] -> w412
                      tunnel: [_ _ w570] -> w408
                      tunnel: w411 -> [_ _ _]
                      tunnel: [w440 _ _] -> w407
                      tunnel: w406 -> [w414 _ w559]
                      frame #0 {
                        w421 = T3."Add Element" ("Action")
                        n241 = Get Date/Time String(want seconds? (F)=TRUE) -> (time string=w439:string)  [unwired: 2 in, 1 out]
                        n242 = local write "Last reading at:"(w439) -> ()
                        n243 = local write "STATUS 1"("Reading LCR meter..." ("status")) -> ()
                        n244 = global read "QC_MeasurementSetup.vi" "CV Measurement Parameters"() -> (w436:T8)
                        n245 = Unbundle By Name(w436) -> ("Temperature Readout"=w416:enum16{"Read Arduino", "Enter manually"}, "Arduino"=w415:refnum<class "ArduinoControl.lvclass">, "LCR"=w430:refnum<class "LCRControl.lvclass">, "AC frequency [Hz]"=w417:i32, "Supply"=w431:refnum<class "SupplyControl.lvclass">, "Set Current Limit?"=w435:bool, "Current Limit [µA]"=w433:dbl)
                        n246 = local read "Current reading No."() -> (w413:u32)
                        n247 = case shown="False" w414 {
                          tunnel: [w456 w478] -> w441
                          tunnel: [w455 w483] -> w437
                          tunnel: w431 -> [w454 w483]
                          tunnel: w430 -> [w453 _]
                          tunnel: [w451 errorcluster {"status"=FALSE, "code"=0, "source"=""} ("error constant")] -> w425
                          tunnel: [w450 w485] -> w423
                          tunnel: [w449 w467] -> w420
                          tunnel: [w448 w486] -> w419
                          tunnel: [w447 w467] -> w418
                          tunnel: w417 -> [w446 _]
                          tunnel: w416 -> [w445 _]
                          tunnel: w415 -> [w444 _]
                          tunnel: w413 -> [_ w476]
                          frame False {
                            n248 = case shown="\"Enter manually\", Default" w445 {
                              tunnel: [w460 w463] -> w448
                              tunnel: [w457 w466] -> w450
                              tunnel: w444 -> [_ w465]
                              frame "Enter manually", Default {
                                n249 = local read "Temp."() -> (w462:dbl[])
                                n250 = local read "RH"() -> (w458:dbl[])
                                n251 = Index Array(array=w462, index=0) -> (element=w460:dbl)
                                n252 = Index Array(array=w458, index=0) -> (element=w457:dbl)
                              }
                              frame "Read Arduino" {
                                n253 = call "ArduinoRead.vi"("Arduino function"=enum16{"T/RH", "Interlock", "Edgesense"}."T/RH", "ArduinoControl in"=w465) -> ("rel. Humidity [%]"=w466:dbl, "Temperature [°C]"=w463:dbl)  [unwired: 4 in, 4 out]
                              }
                            }
                            n254 = call-dynamic "Supply_ReadCurrent.vi"("SupplyControl in"=w454) -> ("error out"=w452:errorcluster, "Current in nA"=w456:dbl, "SupplyControl out"=w455:refnum<class "SupplyControl.lvclass">)  [unwired: 8 in]
                            n255 = call-dynamic "LCR_Readout.vi"("error in (no error)"=w452, "Frequency in Hz"=w446, "LCRControl in"=w453) -> ("error out"=w451:errorcluster, "Resistance in Ohm"=w449:dbl, "Capacitance in pF"=w447:dbl)  [unwired: 5 in, 1 out]
                          }
                          frame True {
                            n256 = local read "Current Volts:"() -> (w473:dbl)
                            n257 = Absolute Value(x=w473) -> (abs(x)=w470:dbl)
                            n258 = Increment(x=w470) -> (x+1=w469:dbl)
                            n259 = Square Root(x=w469) -> (sqrt(x)=w471:dbl)
                            n260 = Random Number (0-1)() -> (number: 0 to 1=w482:dbl)
                            n261 = Exponential(1:w482) -> (0:w481:dbl)
                            n262 = Divide(x=54477.0, y=w471) -> (x/y=w468:dbl)
                            n263 = Add(x=w481, y=w476) -> (x+y=w479:dbl)
                            n264 = Less?(x=w476, y=30) -> (x < y?=w475:bool)
                            n265 = local read "Temp."() -> (w490:dbl[])
                            n266 = local read "RH"() -> (w487:dbl[])
                            n267 = Multiply(x=w479, y=-10.0) -> (x*y=w478:dbl)
                            n268 = Select(t=w468, s=w475, f=3140.0) -> (s? t:f=w467:dbl)
                            n269 = Index Array(array=w490, index=0) -> (element=w486:dbl)
                            n270 = Index Array(array=w487, index=0) -> (element=w485:dbl)
                          }
                        }
                        n271 = Multiply(x=w433, y=1000.0) -> (x*y=w432:dbl)
                        n272 = local read "Current Volts:"() -> (w424:dbl)
                        n273 = case shown="True" w435 {
                          tunnel: w441 -> [_ w495]
                          tunnel: w432 -> [_ w493]
                          tunnel: [FALSE w492] -> w440
                          frame False {
                          }
                          frame True {
                            n274 = Absolute Value(x=w495) -> (abs(x)=w494:dbl)
                            n275 = Greater?(x=w494, y=w493) -> (0:w492:bool)
                          }
                        }
                        n276 = call "CVData.vi"("Action"=w421, "Array No."=u32 3, "Data IN"=w419) -> ()  [unwired: 2 in, 2 out]
                        n277 = call "CVData.vi"("Action"=w421, "Array No."=u32 4, "Data IN"=w423) -> ()  [unwired: 2 in, 2 out]
                        n278 = call "CVData.vi"("Action"=w421, "Array No."=u32 1, "Data IN"=w418) -> ()  [unwired: 2 in, 2 out]
                        n279 = call "CVData.vi"("Action"=w421, "Array No."=u32 2, "Data IN"=w420) -> ()  [unwired: 2 in, 2 out]
                        n280 = call "CVData.vi"("Action"=w421, "Array No."=0, "Data IN"=w424) -> ()  [unwired: 2 in, 2 out]
                        n281 = Increment(x=w413) -> (x+1=w438:u32)
                        n282 = local write "Current reading No."(w438) -> ()
                      }
                      frame #1 {
                        w508 = u32 5 ("y")
                        # "Update plots"
                        n283 = property on="Cgraph" class="WFGraph (strict)"() -> ("YScale.Mapping Mode"=w500:u8)  [unwired: 2 in, 2 out]
                        n284 = call "CVData.vi"("Action"=T3."Read Array", "Array No."=1) -> ("Array OUT"=w497:dbl[])  [unwired: 3 in, 1 out]
                        n285 = property on="Cgraph" class="WFGraph (strict)"("YScale.Minimum"=w500) -> ()  [unwired: 2 in, 2 out]
                        n286 = Greater?(x=w499, y=w508) -> (0:w507:bool)
                        n287 = case shown="True" w507 {
                          tunnel: w499 -> [w516 w519]
                          tunnel: w508 -> [_ w518]
                          tunnel: [w516 w518] -> w506
                          tunnel: [0 w517] -> w504
                          frame False {
                          }
                          frame True {
                            n288 = Subtract(x=w519, y=w518) -> (x-y=w517:u32)
                          }
                        }
                        n289 = Array Subset(array=w497, index=0, length=w499) -> (w503:dbl[])
                        n290 = local read "Cscale"() -> (w509:enum16{"1/C^2 [1/nF^2]", "nF", "pF"})
                        n291 = Absolute Value(x=w503) -> (abs(x)=w502:dbl[])
                        n292 = case shown="..\"1/C^2 [1/nF^2]\"" w509 {
                          tunnel: [w552 w555 w558] -> w514
                          tunnel: w502 -> [w550 w557 w558]
                          frame .."1/C^2 [1/nF^2]" {
                            n293 = Array Size(array=w550) -> (size(s)=w551:i32)
                            n294 = for {
                              N: w551 -> [_]
                              tunnel: w550 -> [w554] mode=indexing
                              tunnel: [w553] -> w552 mode=indexing
                              n295 = formula code="y=1000000./(x*x);"("x"=w554) -> ("y"=w553:dbl)
                            }
                          }
                          frame "nF" {
                            n296 = Divide(x=w557, y=1000.0) -> (x/y=w555:dbl[])
                          }
                          frame "pF".. {
                          }
                        }
                        n297 = for {
                          N: 5 -> [_]
                          tunnel: w506 -> [w525]
                          tunnel: w504 -> [w524]
                          tunnel: w499 -> [w523]
                          i -> [w521]
                          n298 = call "CVData.vi"("Action"=T3."Read Array", "Array No."=w521) -> ("Array OUT"=w520:dbl[])  [unwired: 3 in, 1 out]
                          n299 = case shown="2" w521 {
                            tunnel: w525 -> [w528 w532 w537 _ _]
                            tunnel: w524 -> [w529 w533 w538 _ _]
                            tunnel: w520 -> [w527 w531 w539 w543 w548]
                            tunnel: w523 -> [_ _ _ w541 w546]
                            frame ..0 {
                              n300 = Array Subset(array=w527, index=w529, length=w528) -> (w526:dbl[])
                              n301 = local write "Volts"(w526) -> ()
                            }
                            frame 1 {
                              n302 = Array Subset(array=w531, index=w533, length=w532) -> (w530:dbl[])
                              n303 = local write "Capacitance"(w530) -> ()
                            }
                            frame 2 {
                              n304 = Array Subset(array=w539, index=w538, length=w537) -> (w536:dbl[])
                              n305 = Multiply(x=w536, y=0.001) -> (x*y=w535:dbl[])
                              n306 = local write "Resistance"(w535) -> ()
                            }
                            frame 3 {
                              n307 = Decrement(x=w541) -> (x-1=w540:u32)
                              n308 = Array Subset(array=w543, index=w540, length=1) -> (w542:dbl[])
                              n309 = local write "Temp."(w542) -> ()
                            }
                            frame 4.. {
                              n310 = Decrement(x=w546) -> (x-1=w545:u32)
                              n311 = Array Subset(array=w548, index=w545, length=1) -> (w547:dbl[])
                              n312 = local write "RH"(w547) -> ()
                            }
                          }
                        }
                        n313 = local read "Initial volts [V]"() -> (w512:dbl)
                        n314 = Absolute Value(x=w511) -> (abs(x)=w510:dbl)
                        n315 = Bundle("Initial volts [V]"=w512, w510, w514) -> (w501:cluster{"Initial volts [V]":dbl, dbl, dbl[]})  [unwired: 1 in]
                        n316 = local write "Cgraph"(w501) -> ()
                      }
                      frame #2 {
                        # "Increment volts and check for end of loop"
                        n317 = local read "positive ramp?"() -> (w569:bool)
                        n318 = local read "Current Volts:"() -> (w565:dbl)
                        n319 = case shown="True" w569 {
                          tunnel: w564 -> [w576 w580]
                          tunnel: w573 -> [w577 w583]
                          tunnel: [w575 w582] -> w560
                          tunnel: [w574 w579] -> w572
                          tunnel: w565 -> [w578 w581]
                          frame False {
                            n320 = Subtract(x=w578, y=w577) -> (x-y=w574:dbl)
                            n321 = Greater Or Equal?(x=w574, y=w576) -> (x >= y?=w575:bool)
                          }
                          frame True {
                            n322 = Add(x=w581, y=w583) -> (x+y=w579:dbl)
                            n323 = Less Or Equal?(x=w579, y=w580) -> (x <= y?=w582:bool)
                          }
                        }
                        n324 = Quotient & Remainder(x=w565, y=w564) -> (x-y*floor(x/y)=w566:dbl, floor(x/y)=w563:dbl)
                        n325 = Not Equal To 0?(x=w566) -> (x != 0?=w561:bool)
                        n326 = Equal To 0?(x=w563) -> (x = 0?=w562:bool)
                        n327 = Or(x=w561, y=w562) -> ()  [unwired: 1 out]
                        n328 = case shown="True" w560 {
                          tunnel: w572 -> [_ w593]
                          tunnel: [TRUE FALSE] -> w571
                          tunnel: [FALSE w594] -> w570
                          tunnel: w565 -> [_ w592]
                          tunnel: w568 -> [_ w591]
                          tunnel: w567 -> [_ w590]
                          tunnel: w559 -> [_ w586]
                          frame False {
                          }
                          frame True {
                            n329 = case shown="True" w586 {
                              tunnel: [w604 FALSE] -> w594
                              tunnel: w593 -> [w603 w605]
                              tunnel: w592 -> [w602 _]
                              tunnel: w591 -> [w601 w606]
                              tunnel: w590 -> [w600 _]
                              tunnel: [w599 w605] -> w589
                              tunnel: [w596 w606] -> w588
                              frame False {
                                n330 = local read "step [V]"() -> (w598:dbl)
                                n331 = call "SupplyRamp.vi"("error in"=w601, "Requested Voltage"=w603, "Step Size"=w598, "Step Delay"=100, "Supply IN"=w600, "Starting Voltage"=w602) -> ("error out"=w596:errorcluster, "Compliance exceeded"=w604:bool, "Current Voltage"=w599:dbl)  [unwired: 2 in, 1 out]
                              }
                              frame True {
                              }
                            }
                            n332 = local write "STATUS 1"("Incrementing volts.") -> ()
                            n333 = case shown="No Error" w588 {
                              tunnel: w589 -> [w608 _]
                              frame No Error {
                                n334 = local write "Current Volts:"(w608) -> ()
                              }
                              frame Error {
                              }
                            }
                            n335 = property on="Bias On/Off:" class="Bool (strict)"("Blinking"=w594) -> ()  [unwired: 2 in, 2 out]
                          }
                        }
                      }
                    }
                  }
                  frame True {
                    w609 = FALSE
                  }
                }
              }
            }
            n336 = case shown="True" w310 {
              frame False {
              }
              frame True {
                n337 = property on="Bias On/Off:" class="Bool (strict)"("Blinking"=TRUE) -> ()  [unwired: 2 in, 2 out]
              }
            }
            n338 = Build Array(w312, w310, "abort", w311) -> (w316:bool[])
            n339 = Or Array Elements(Boolean array=w316) -> (logical OR=w322:bool)
            n340 = Not(x=w322) -> (.not. x?=w321:bool)
          }
        }
        frame True {
          w611 = FALSE
          # "compliance was exceeded when first voltage applied."
          # "Flag compliance as reason for end of run"
          n341 = local write "STATUS 1"("Run aborted - compliance exceeded.") -> ()
          n342 = Build Array(w611, TRUE, w611, w611) -> (w612:bool[])
        }
      }
      n343 = Search 1D Array(1D array=w297, element=TRUE) -> (index of element=w295:i32)  [unwired: 1 in]
      n344 = Increment(x=w295) -> (x+1=w294:i32)
      n345 = case shown="..0" w294 {
        tunnel: ["" "Run ended normally" "Compliance exceeded" "Run aborted - by user" "Run aborted - Ilimit exceeded"] -> w289
        frame ..0 {
        }
        frame 1 {
        }
        frame 2 {
          # "Determine reason for end of run."
        }
        frame 3 {
        }
        frame 4.. {
        }
      }
      n346 = global read "QC_RunInformation.vi" "Run info"() -> (w293:T7)
      n347 = Bundle By Name(cluster=w293, "End of Run comment:"=w289) -> (w288:T7)
      n348 = global write "QC_RunInformation.vi" "Run info"(w288) -> ()
      n349 = Concatenate Strings(w289, "\r\n", "RAMPING DOWN VOLTS") -> (w292:string)
      n350 = local write "STATUS 1"(w292) -> ()
    }
    frame #4 {
      # "Ramp down and switch off supply"
      n351 = stacked-sequence {
        tunnel: w615 -> [w616 _ _]
        frame #0 {
          # "Tie up loose ends. Set volts to zero and switch to standby"
          n352 = global read "QC_MeasurementSetup.vi" "CV Measurement Parameters"() -> (w622:T8)
          n353 = Unbundle By Name(w622) -> ("Supply"=w619:refnum<class "SupplyControl.lvclass">, "Ramp down steps [V]"=w621:dbl, "Ramp down Interval [s]"=w620:i32, "Measurement switch"=w618:refnum<class "Switching.lvclass">, "Measurement switch used?"=w617:bool)
          n354 = case shown="False" w616 {
            tunnel: 0.0 -> [w636 w645]
            tunnel: [w635 w645] -> w623
            tunnel: w621 -> [w632 _]
            tunnel: w620 -> [w631 _]
            tunnel: w619 -> [w630 _]
            tunnel: w618 -> [w626 _]
            tunnel: w617 -> [w625 _]
            frame False {
              # "Ramp down volts now"
              n355 = Multiply(x=w631, y=1000) -> (x*y=w634:i32)
              n356 = local read "Current Volts:"() -> (w637:dbl)
              n357 = call "SupplyRamp.vi"("Requested Voltage"=w636, "Step Size"=w632, "Step Delay"=w634, "Supply IN"=w630, "Starting Voltage"=w637) -> ("error out"=w628:errorcluster, "Supply OUT"=w629:refnum<class "SupplyControl.lvclass">, "Current Voltage"=w635:dbl)  [unwired: 3 in, 1 out]
              n358 = stacked-sequence {
                tunnel: w629 -> [_ w641]
                tunnel: w628 -> [_ w640]
                tunnel: [_ w639] -> w627
                frame #0 {
                  n359 = Wait (ms)(milliseconds to wait=5000) -> ()  [unwired: 1 out]
                }
                frame #1 {
                  n360 = call-dynamic "Supply_Stby.vi"("error in (no error)"=w640, "SupplyControl in"=w641) -> ("error out"=w639:errorcluster)  [unwired: 8 in, 1 out]
                }
              }
              n361 = case shown="True" w625 {
                tunnel: w626 -> [_ w644]
                tunnel: w627 -> [_ w643]
                frame False {
                }
                frame True {
                  n362 = call-dynamic "MatrixSwitch.vi"("error in (no error)"=w643, "Action"=T4."Reset", "Switching in"=w644) -> ()  [unwired: 6 in, 3 out]
                }
              }
            }
            frame True {
            }
          }
          n363 = local write "Current Volts:"(w623) -> ()
        }
        frame #1 {
          w650 = 0
          n364 = local write "Bias On/Off:"(FALSE ("Visible")) -> ()
          n365 = local write "Current Volts:"(0.0 ("Current Volts:")) -> ()
          n366 = property on="abort" class="Bool (strict)"("DisabledEnum"=2) -> ()  [unwired: 2 in, 2 out]
          n367 = property on="Quit & Save" class="Bool"("DisabledEnum"=w650) -> ()  [unwired: 2 in, 2 out]
          n368 = property on="quit (no save)" class="Bool"("DisabledEnum"=w650) -> ()  [unwired: 2 in, 2 out]
          n369 = local write "STATUS 1"("Run finished. \nSave data?" ("STATUS 1")) -> ()
        }
        frame #2 {
          n370 = Current VI's Path() -> (path=w652:path)
          n371 = call "SaveJPEG.vi"("Test"="CV", "File Path Control"=w652) -> ()  [unwired: 1 in, 2 out]
        }
      }
    }
    frame #5 {
      # "Loop and await decision on whether to save or junk data"
      # "Display and save data"
      n372 = case shown="False" w653 {
        frame False {
          n373 = global read "QC_MeasurementSetup.vi" "CV Measurement Parameters"() -> (w668:T8)
          n374 = Unbundle By Name(w668) -> ("Temperature Readout"=w667:enum16{"Read Arduino", "Enter manually"}, "Arduino"=w666:refnum<class "ArduinoControl.lvclass">)
          n375 = case shown="\"Read Arduino\"" w667 {
            tunnel: w666 -> [_ w669]
            frame "Enter manually", Default {
            }
            frame "Read Arduino" {
              n376 = call "ArduinoClose.vi"("ArduinoControl in"=w669) -> ()  [unwired: 9 in, 2 out]
            }
          }
        }
        frame True {
        }
      }
      n377 = local read "Scales"() -> (w662:T1)
      n378 = local read "Cscale"() -> (w661:enum16{"1/C^2 [1/nF^2]", "nF", "pF"})
      n379 = while {
        shift-left: w661 -> [w713]
        shift-right: [w712] -> _
        shift-left: w662 -> [w715]
        shift-right: [w714] -> _
        tunnel: ["Quit & Save"] -> w664
        tunnel: ["quit (no save)"] -> w663
        stop <- w710 continue-if-true
        n380 = local read "Cscale"() -> (w712:enum16{"1/C^2 [1/nF^2]", "nF", "pF"})
        n381 = local read "Scales"() -> (w714:T1)
        n382 = Not Equal?(x=w715, y=w714) -> (x != y?=w708:bool)
        n383 = Not Equal?(x=w713, y=w712) -> (x != y?=w707:bool)
        n384 = case shown="True" w708 {
          tunnel: w714 -> [_ w742]
          frame False {
          }
          frame True {
            n385 = case shown="..\"Lin - Lin\"" w742 {
              tunnel: [w743 1 0 w748] -> w741
              tunnel: [w743 0 1 w748] -> w740
              frame .."Lin - Lin" {
                w743 = 0
              }
              frame "Log - Lin" {
              }
              frame "Lin - Log" {
              }
              frame "Log - log".. {
                w748 = 1
              }
            }
            n386 = property on="Cgraph" class="WFGraph (strict)"("X Scale.Mapping Mode"=w741) -> ()  [unwired: 2 in, 2 out]
            n387 = property on="Cgraph" class="WFGraph (strict)"("Y Scale.Mapping Mode"=w740, "YScale.Minimum"=w740) -> ()  [unwired: 2 in, 2 out]
          }
        }
        n388 = case shown="True" w707 {
          tunnel: w712 -> [_ w720]
          frame False {
          }
          frame True {
            n389 = property on="Cgraph" class="WFGraph (strict)"() -> ("YScale.Mapping Mode"=w723:u8)  [unwired: 2 in, 2 out]
            n390 = property on="Cgraph" class="WFGraph (strict)"("YScale.Minimum"=w723) -> ()  [unwired: 2 in, 2 out]
            n391 = global read "QC_MeasurementSetup.vi" "CV Measurement Parameters"() -> (w722:T8)
            n392 = Unbundle By Name(w722) -> ("Initial Voltage [V]"=w725:dbl, "Step Size [V]"=w727:dbl, "Number Of Steps"=w724:u32)
            n393 = call "CVData.vi"("Action"=T3."Read Array", "Array No."=u32 1 ("Action")) -> ("Array OUT"=w716:dbl[])  [unwired: 3 in, 1 out]
            n394 = Absolute Value(x=w727) -> (abs(x)=w726:dbl)
            n395 = Array Subset(array=w716, index=0, length=w724) -> (w728:dbl[])
            n396 = Absolute Value(x=w728) -> (abs(x)=w721:dbl[])
            n397 = case shown="..\"1/C^2 [1/nF^2]\"" w720 {
              tunnel: [w733 w736 w739] -> w719
              tunnel: w721 -> [w731 w738 w739]
              frame .."1/C^2 [1/nF^2]" {
                n398 = Array Size(array=w731) -> (size(s)=w732:i32)
                n399 = for {
                  N: w732 -> [_]
                  tunnel: w731 -> [w735] mode=indexing
                  tunnel: [w734] -> w733 mode=indexing
                  n400 = formula code="y=1000000./(x*x);"("x"=w735) -> ("y"=w734:dbl)
                }
              }
              frame "nF" {
                n401 = Divide(x=w738, y=1000.0) -> (x/y=w736:dbl[])
              }
              frame "pF".. {
              }
            }
            n402 = Bundle("Initial Voltage [V]"=w725, w726, w719) -> (w729:cluster{"Initial Voltage [V]":dbl, dbl, dbl[]})  [unwired: 1 in]
            n403 = local write "Cgraph"(w729) -> ()
          }
        }
        n404 = local read "Run uninterrupted?"() -> (w706:bool)
        n405 = Compound Arithmetic op=OR("Quit & Save", "quit (no save)", w706) -> (invert w710:bool)
      }
      n406 = case shown="True" w663 {
        tunnel: [FALSE w750] -> w665
        frame False {
        }
        frame True {
          n407 = Two Button Dialog(message="Are you sure you don't want to save the data?", 1:"Quit" ("F button name (\"Cancel\")"), 2:"Save data" ("T button name (\"OK\")")) -> (T button?=w750:bool)
        }
      }
      n408 = local read "Run uninterrupted?"() -> (w654:bool)
      n409 = Compound Arithmetic op=OR(w664, w665, w654) -> (w660:bool)
      n410 = flat-sequence {
        tunnel: w660 -> [w672]
        tunnel: [w672] -> w656
        tunnel: [TRUE] -> w655
        tunnel: w654 -> [w670]
        frame #0 {
          n411 = case shown="True" w672 {
            tunnel: ["" w705] -> w682
            tunnel: [_ w691] -> w680
            tunnel: w670 -> [_ w684]
            frame False {
            }
            frame True {
              w689 = T3."Read Array" ("Action")
              n412 = local write "STATUS 1"("Saving Data ...") -> ()
              n413 = call "CVData.vi"("Action"=w689, "Array No."=u32 2 ("Action")) -> ("Array OUT"=w687:dbl[])  [unwired: 3 in, 1 out]
              n414 = call "CVData.vi"("Action"=w689, "Array No."=u32 4 ("Action")) -> ("Array OUT"=w702:dbl[])  [unwired: 3 in, 1 out]
              n415 = call "CVData.vi"("Action"=w689, "Array No."=u32 3 ("Action")) -> ("Array OUT"=w701:dbl[])  [unwired: 3 in, 1 out]
              n416 = call <vilib>:"Std Deviation and Variance.vi"("X"=w702) -> ("mean"=w692:dbl)  [unwired: 1 in, 2 out]
              n417 = call <vilib>:"Std Deviation and Variance.vi"("X"=w701) -> ("mean"=w693:dbl)  [unwired: 1 in, 2 out]
              n418 = Multiply(x=w687, y=0.001) -> (x*y=w686:dbl[])
              n419 = call "CVData.vi"("Action"=w689, "Array No."=u32 0 ("Action")) -> ("Array OUT"=w696:dbl[])  [unwired: 3 in, 1 out]
              n420 = call "CVData.vi"("Action"=w689, "Array No."=u32 1 ("Action")) -> ("Array OUT"=w695:dbl[])  [unwired: 3 in, 1 out]
              n421 = call "SaveDataFile.vi"("Temperature"=w693, "Run uninterrupted?"=w684, "Humidity"=w692, "Array Titles"="Voltage[V] Capacitance[pF] Resistance[kOhm]", "Strip Segment"="") -> ("Path + Filename OUT"=w705:string, "Error Out"=w691:errorcluster)  [unwired: 7 in, 2 out]
              n422 = Build Array(w696, w695, w686) -> (w694:dbl[][])
              n423 = Transpose 2D Array(2D array=w694) -> ()  [unwired: 1 out]
            }
          }
          n424 = global read "QC_MeasurementSetup.vi" "CV Measurement Parameters"() -> (w681:T8)
          n425 = Unbundle By Name(w681) -> ("V_depletion Limit [V]"=w674:dbl)
          n426 = call "ScanFeedback.vi"("measurement type"=T5."CV") -> ("V depletion"=w676:dbl)  [unwired: 4 in, 4 out]
          n427 = Absolute Value(x=w676) -> (abs(x)=w675:dbl)
          n428 = Absolute Value(x=w674) -> (abs(x)=w673:dbl)
          n429 = Less Or Equal?(x=w675, y=w673) -> (x <= y?=w677:bool)
          n430 = call "WriteLogFile.vi"("Run uninterrupted?"=w670, "Automatic warning"="", "Data File"=w682, "Error In"=w680, "DUT passed?"=w677, "Value TechSpec criteria"=w676, "Files saved?"=w672) -> ()  [unwired: 4 in, 1 out]
        }
      }
      n431 = Select(t="Run finished.\nData saved." ("STATUS 1"), s=w656, f="Run finished.\nData not saved." ("STATUS 1")) -> (s? t:f=w659:string)
      n432 = local write "STATUS 1"(w659) -> ()
      "Done!" <- w655
    }
  }
